vi "tearDown.vi"(8 "error in":errorcluster, 11 "reference in":refnum<class "Create Execution Unit.lvclass">) -> (0 "error out":errorcluster, 3 "reference out":refnum<class "Create Execution Unit.lvclass">)   [LabVIEW 2020, in "Create Execution Unit.lvclass"]
doc: "tearDown runs after the test method has completed. Use this method to clean up any operations or references that were opened by setUp or the test method. Unit tests should be independent of other unit tests so this VI should ensure that the next test can run in a 'clean' test environment."
uses:
  Create Execution Unit.lvclass
  niveristand-custom-device-testing-tools/VeriStandTestUtilities/VeriStandTestUtilities.lvlib
  niveristand-custom-device-testing-tools/VeriStandScriptingTestCase/VeriStandScriptingTestCase.lvclass
  C:/Git/niveristand-custom-device-testing-tools/VeriStandScriptingTestCase/VeriStandScriptingTestCase.lvclass
  C:/Program Files (x86)/National Instruments/LabVIEW 2020/vi.lib/addons/_JKI Toolkits/VI Tester/TestCase.llb/TestCase.lvclass
  C:/Git/niveristand-ballard-milStd1553-custom-device/Source/Custom Device Support/Tests/Unit/Create Execution Unit/Create Execution Unit.lvclass
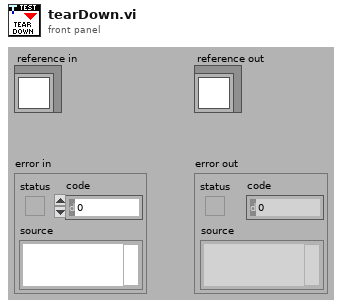
[diagram p1: front panel]
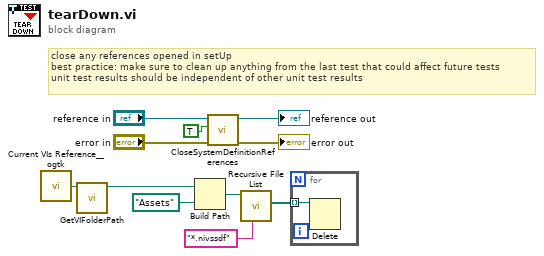
[diagram p0: block diagram]
diagram:
  # "close any references opened in setUp\nbest practice: make sure to clean up anything from the last test that could affect future tests\nunit test results should be independent of other unit test results"
  n1 = call <userlib>:"Current VIs Reference__ogtk.vi"() -> ("Current VI's reference"=w11:refnum<vi>)  [unwired: 5 in]
  n2 = call "GetVIFolderPath.vi"("VI Reference in"=w11) -> ("VI Folder Path out"=w10:path)  [unwired: 9 in, 1 out]
  n3 = Build Path(base path=w10, name or relative path=path "Assets") -> (appended path=w8:path)
  n4 = call "CloseSystemDefinitionReferences.vi"("error in"="error in", "Delete Sysdef? (F)"=TRUE, "VeriStandScriptingTestCase in"="reference in") -> ("error out"=→"error out":errorcluster, "VeriStandScriptingTestCase out"=→"reference out":refnum<class "Create Execution Unit.lvclass">)  [unwired: 7 in]
  n5 = call <vilib>:"Recursive File List.vi"("pattern"="*.nivssdf", "Folder Path"=w8) -> ("All Files in Dir"=w6:path[])  [unwired: 5 in, 4 out]
  n6 = for {
    tunnel: w6 -> [w12] mode=indexing
    n7 = Delete(path (use dialog)=w12) -> ()  [unwired: 4 in, 3 out]
  }
